vi "Actualiza Contador.vi"(8 "error in (no error)":errorcluster, 10 "Contador":dbl, 11 "Contador in":refnum<class "Contador.lvclass">) -> (0 "error out":errorcluster, 3 "Contador out":refnum<class "Contador.lvclass">)   [LabVIEW 2020, in "Contador.lvlib" / "Contador.lvclass"]
uses:
  Contador.lvclass
  Contador.lvclass/Contador.ctl
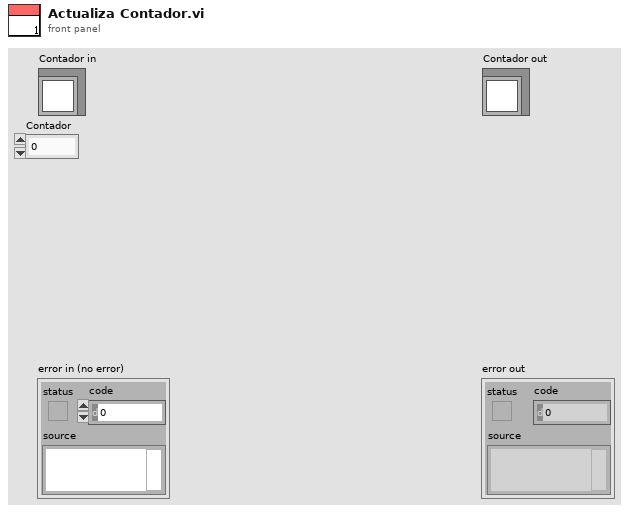
[diagram p1: front panel]
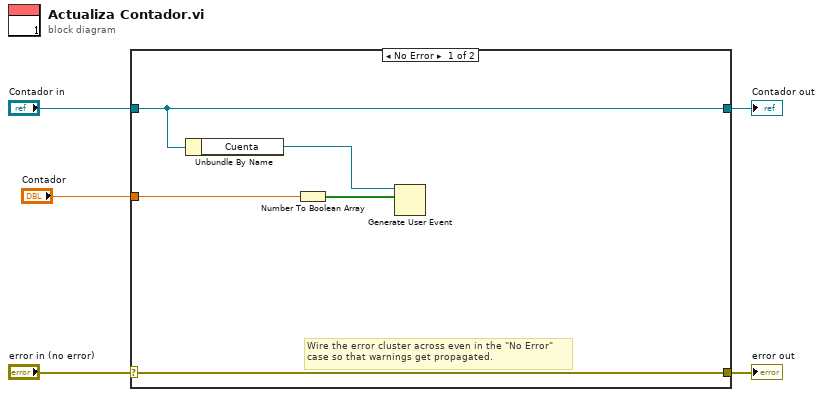
[diagram p0: block diagram]
diagram:
  n1 = case shown="No Error" "error in (no error)" {
    selector: "error in (no error)" -> [w10 w12]
    tunnel: [w10 w12] -> w4
    tunnel: [w9 w11] -> w2
    tunnel: "Contador in" -> [w9 w11]
    tunnel: "Contador" -> [w6 _]
    frame No Error {
      # "Wire the error cluster across even in the \"No Error\"\ncase so that warnings get propagated."
      n2 = Unbundle By Name(w9) -> ("Cuenta"=w8:refnum<user-event>)
      n3 = Number To Boolean Array(number=w6) -> (Boolean array=w7:bool[])
      n4 = Generate User Event(user event=w8, event data cluster=w7) -> ()  [unwired: 2 in, 2 out]
    }
    frame Error {
    }
  }
  "error out" <- w4
  "Contador out" <- w2
